vi "Salman's Tip Tester.vi"() -> ()   [LabVIEW 2016]
uses:
  <instrlib>/Stanford Research 830/Public/Data/Read (All Parameters).vi
  <vilib>/Analysis/1siggen.llb/Ramp Pattern by Delta.vi
  <vilib>/express/express shared/transition.llb/Dynamic To Waveform Array.vi
  <vilib>/express/express signal manip/GetorSetDDTAttributes/Set DDT Attributes/SetT0.vi
  <vilib>/express/express shared/transition.llb/Waveform Array To Dynamic.vi
  <vilib>/express/express signal manip/GetorSetDDTAttributes/Set DDT Attributes/Set DDT Properties.xnode
  <vilib>/Analysis/NI_AALBase.lvlib
  <instrlib>/Stanford Research 830/Stanford Research 830.lvlib
  <instrlib>/Agilent 3352X Series/Agilent 3352X Series.lvlib
panel:
  out "Reference Frequency":dbl
  in  "stop":bool
  out "Y-Value":dbl
  out "X-Value":dbl
  in  "?":T1(tab)
  in  "Lock In":refnum<visa-resource-name>
  in  "Frequency Generator":refnum<visa-resource-name>
  in  "Sensitivity":i16(ring)=-1 items=["Auto Gain"=-1, "2 nV/fA"=0, "5 nV/fA"=1, "10 nV/fA"=2, "20 nV/fA"=3, "50 nV/fA"=4, "100 nV/fA"=5, "200 nV/fA"=6, "500 nV/fA"=7, "1 uV/pA"=8, "2 uV/pA"=9, "5 uV/pA"=10, "10 uV/pA"=11, "20 uV/pA"=12, "50 uV/pA"=13, "100 uV/pA"=14, "200 uV/pA"=15, "500 uV/pA"=16, "1 mV/nA"=17, "2 mV/nA"=18, "5 mV/nA"=19, "10 mV/nA"=20, "20 mV/nA"=21, "50 mV/nA"=22, "100 mV/nA"=23, "200 mV/nA"=24, "500 mV/mA"=25, "1 V/uA"=26]
  in  "Auto Phase":bool=TRUE
  in  "Lock In Frequency (Hz)":dbl=1000.0
  in  "Lock In Output (V)":dbl=1.0
  in  "External Reference Trigger":u16(ring) items=["Sine Zero Crossing", "TTL Rising Edge", "TTL Falling Edge"]
  in  "Reference Source":u16(ring)=1 items=["External", "Internal"]
  in  "Amplitude (V)":dbl=0.1
  in  "Waveform Function":i32(ring) items=["Sine"=0, "Square"=1, "Ramp"=2, "Noise"=3, "DC"=4, "Triangle"=5, "Pulse"=6, "Sinc"=11, "D-Lorentz"=12, "Gaussian"=13, "Expo Fall"=14, "Expo Rise"=15, "Haversine"=16]
  in  "Frequency (Hz)":dbl=1000.0
  in  "Save File Name":path=path "G:/UCB/Instruments/tip making/Qplus AFM tip making/qplus test/Caihong/CJ39.xlsx" caption="Filename"
  out "Frequency (Hz) 2":dbl
  out "XY Graph 3":cluster{dbl[], dbl[]}[](graph) caption="XY Graph 2"
  out "XY Graph 2":cluster{dbl[], dbl[]}[](graph)
  in  "Start Sweep":bool
  in  "Wait Time (s)":dbl
  in  "Step Size (Hz)":dbl
  in  "Final Frequency":dbl
  in  "Start Frequency":dbl
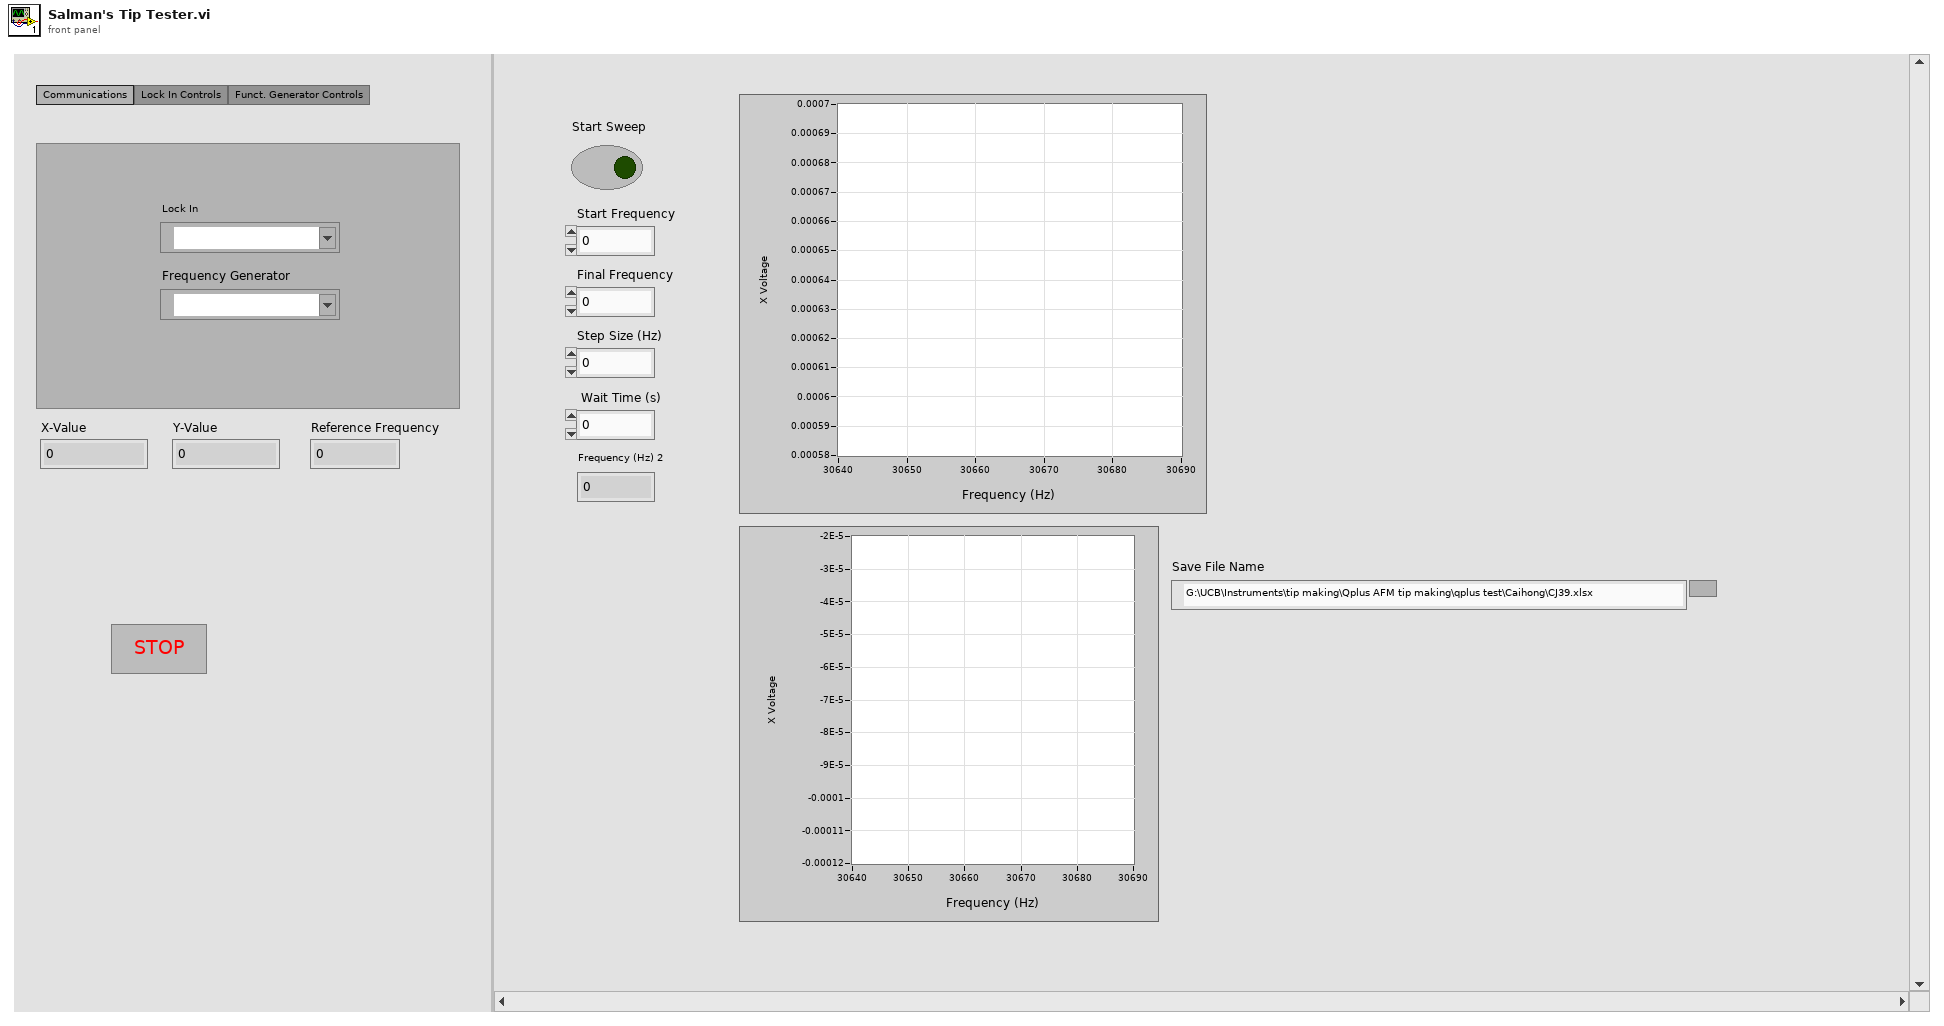
[diagram p1: front panel]
types:
  T1 = enum32{"Communications", "Lock In Controls", "Funct. Generator Controls"}
  T2 = cluster{"X-Value":dbl, "Y-Value":dbl, "R-Value":dbl, "Theta-Value":dbl, "Aux In 1 Value":dbl, "Aux In 2 Value":dbl, "Aux In 3 Value":dbl, "Aux In 4 Value":dbl, "Reference Frequency":dbl, "Channel 1 Display":dbl, "Channel 2 Display":dbl}
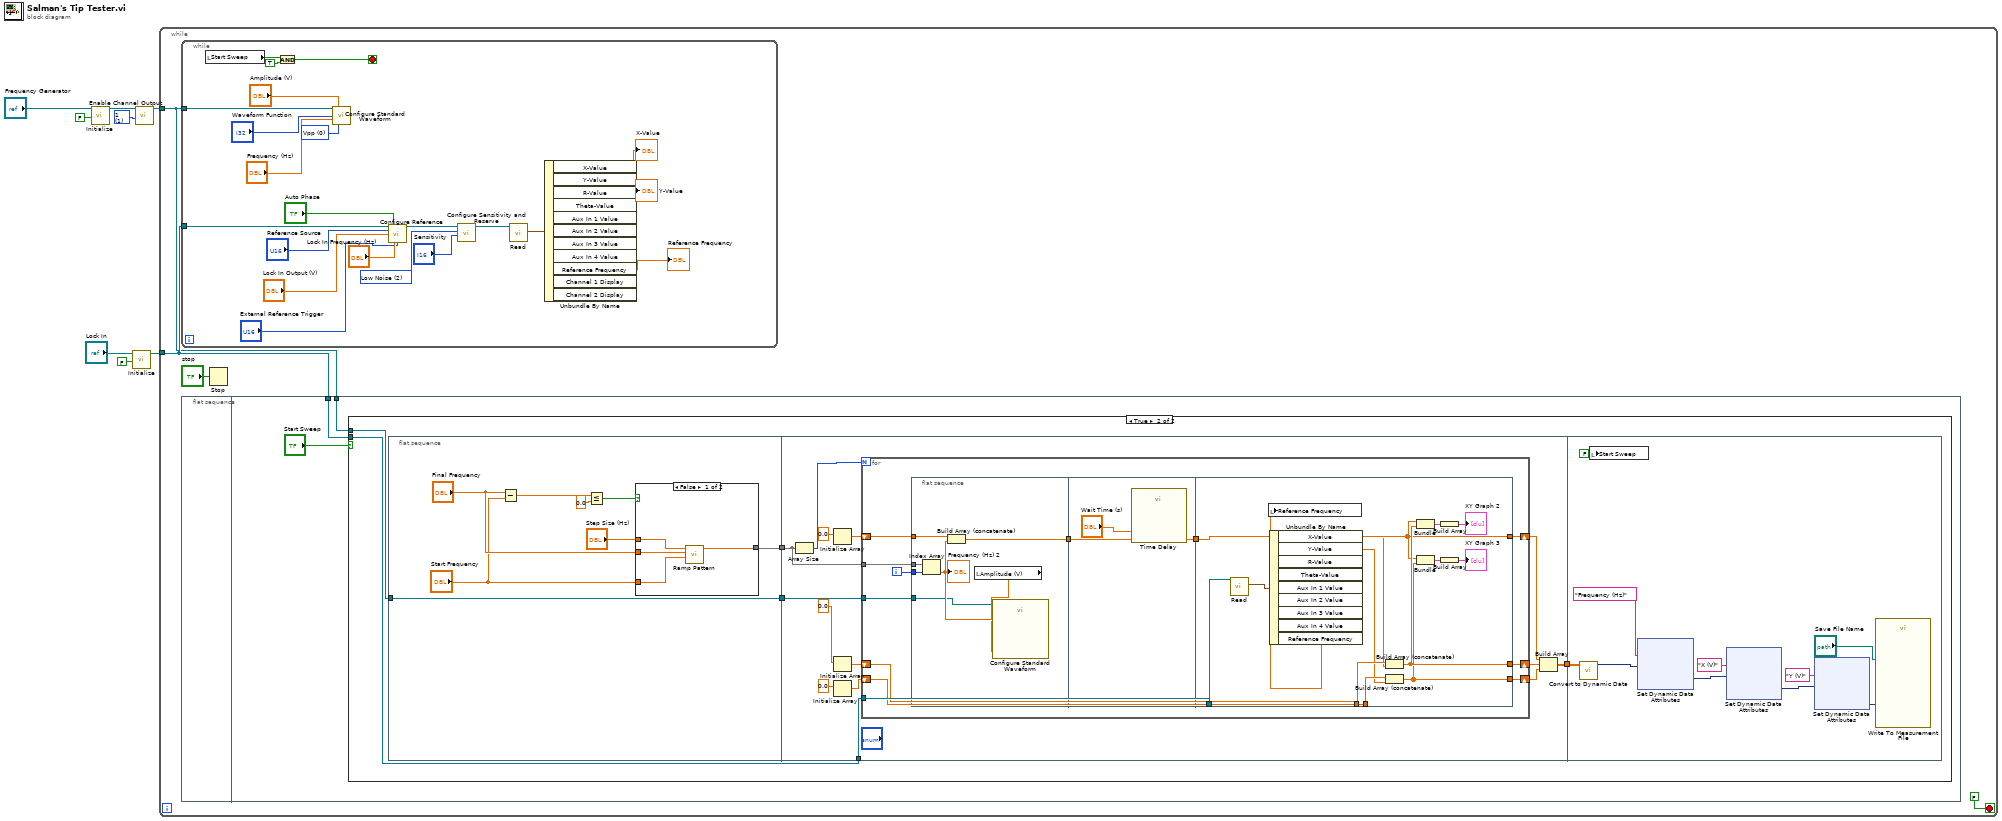
[diagram p0: block diagram]
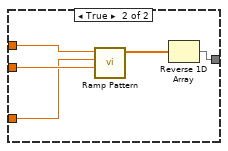
[diagram p3: hidden frame]
diagram:
  w3 = u16 1 items=["1"=1, "2"=2] ("Channel (1: 1)")
  n1 = call <instrlib>:"Initialize.vi"("Reset (Enable)"=FALSE ("Reset (True)"), "VISA resource name"="Frequency Generator") -> ("VISA resource name out"=w2:refnum<visa-resource-name>)  [unwired: 8 in, 1 out]
  n2 = call <instrlib>:"Initialize.vi"("Reset (True)"=FALSE, "VISA resource name"="Lock In") -> ("VISA resource name out"=w7:refnum<visa-resource-name>)  [unwired: 8 in, 1 out]
  n3 = call <instrlib>:"Enable Channel Output.vi"("Channel (1: 1)"=w3, "VISA resource name"=w2) -> ("VISA resource name out"=w1:refnum<visa-resource-name>)  [unwired: 8 in, 1 out]
  n4 = while {
    tunnel: w7 -> [w12]
    tunnel: w1 -> [w9]
    stop <- FALSE stop-if-true
    n5 = while {
      tunnel: w12 -> [w160]
      tunnel: w9 -> [w143]
      stop <- w154 stop-if-true
      w144 = 0 items=["Vpp", "VRMS", "DBM"] ("Amplitude Unit (0: Vpp)")
      w152 = i16 2 items=["Auto Reserve"=-1, "High Reserve"=0, "Normal"=1, "Low Noise"=2] ("Dynamic Reserve (-1: Auto Reserve)")
      n6 = local read "Start Sweep"() -> (w156:bool)
      n7 = And(x=w156, y=TRUE) -> (x .and. y?=w154:bool)
      n8 = call <instrlib>:"Configure Standard Waveform.vi"("VISA resource name"=w143, "Amplitude (0.1 Vpp)"="Amplitude (V)", "Waveform Function (0: Sine)"="Waveform Function", "Frequency/Sample Rate/Bandwidth (1000 Hz)"="Frequency (Hz)", "Amplitude Unit (0: Vpp)"=w144) -> ()  [unwired: 9 in, 2 out]
      n9 = call "Configure Reference.vi"("VISA resource name"=w160, "Auto Phase (T: Enabled)"="Auto Phase", "Reference Source (1: Internal)"="Reference Source", "Sine Output Amplitude (1 V)"="Lock In Output (V)", "Internal Reference Frequency (1000 Hz)"="Lock In Frequency (Hz)", "External Reference Trigger (0: Sine Zero Crossing)"="External Reference Trigger") -> ("VISA resource name out"=w153:refnum<visa-resource-name>)  [unwired: 8 in, 1 out]
      n10 = call <instrlib>:"Configure Sensitivity and Reserve.vi"("Sensitivity (-1: Auto gain)"="Sensitivity", "Dynamic Reserve (-1: Auto Reserve)"=w152, "VISA resource name"=w153) -> ("VISA resource name out"=w150:refnum<visa-resource-name>)  [unwired: 7 in, 1 out]
      n11 = call-poly <instrlib>:"Read.vi"("VISA resource name"=w150) -> ("Parameter Values"=w142:T2)  [unwired: 8 in, 2 out]
      n12 = Unbundle By Name(w142) -> ("X-Value"=→"X-Value":dbl, "Y-Value"=→"Y-Value":dbl, "Reference Frequency"=→"Reference Frequency":dbl)  [unwired: 8 out]
    }
    n13 = flat-sequence {
      tunnel: w12 -> [w14]
      tunnel: w9 -> [w13]
      frame #0 {
      }
      frame #1 {
        n14 = case shown="True" "Start Sweep" {
          tunnel: w14 -> [_ w19]
          tunnel: w13 -> [_ w18]
          frame False {
          }
          frame True {
            n15 = flat-sequence {
              tunnel: [w23] -> w20
              tunnel: w18 -> [w21]
              tunnel: [w21] -> w17
              tunnel: w20 -> [w51]
              tunnel: w19 -> [w47]
              tunnel: w17 -> [w44]
              tunnel: [w38] -> w16
              tunnel: w16 -> [w95]
              frame #0 {
                n16 = Subtract(x="Final Frequency", y="Start Frequency") -> (x-y=w28:dbl)
                n17 = Less Or Equal?(x=w28, y=0.0) -> (x <= y?=w26:bool)
                n18 = case shown="False" w26 {
                  tunnel: "Final Frequency" -> [w32 w34]
                  tunnel: "Start Frequency" -> [w31 w33]
                  tunnel: "Step Size (Hz)" -> [w30 w37]
                  tunnel: [w29 w35] -> w23
                  frame False {
                    n19 = call-poly <vilib>:"Ramp Pattern.vi"("start"=w31, "end"=w32, "delta"=w30) -> ("Ramp Pattern"=w29:dbl[])  [unwired: 6 in, 2 out]
                  }
                  frame True {
                    n20 = call-poly <vilib>:"Ramp Pattern.vi"("start"=w34, "end"=w33, "delta"=w37) -> ("Ramp Pattern"=w36:dbl[])  [unwired: 6 in, 2 out]
                    n21 = Reverse 1D Array(array=w36) -> (reversed array=w35:dbl[])
                  }
                }
              }
              frame #1 {
                n22 = Array Size(array=w51) -> (size(s)=w49:i32)
                n23 = Initialize Array(0.0 ("element")) -> (w48:dbl[])  [unwired: 1 in]
                n24 = Initialize Array(0.0 ("element")) -> (w45:dbl[])  [unwired: 1 in]
                n25 = Initialize Array(0.0 ("element")) -> (w42:dbl[])  [unwired: 1 in]
                n26 = for {
                  N: w49 -> [_]
                  tunnel: w51 -> [w61]
                  shift-right: [w60] -> w39
                  shift-left: w48 -> [w63]
                  tunnel: w47 -> [w57]
                  shift-right: [w56] -> w41
                  shift-left: w45 -> [w55]
                  tunnel: w44 -> [w54]
                  shift-right: [w52] -> w40
                  shift-left: w42 -> [w53]
                  i -> [w62]
                  n27 = flat-sequence {
                    tunnel: w63 -> [w70]
                    tunnel: w62 -> [w69]
                    tunnel: w61 -> [w68]
                    tunnel: [w67] -> w58
                    tunnel: w54 -> [w64]
                    tunnel: [w71] -> w59
                    tunnel: w58 -> [w71]
                    tunnel: [w76] -> w60
                    tunnel: w59 -> [w76]
                    tunnel: w57 -> [w74]
                    tunnel: w55 -> [w85]
                    tunnel: [w84] -> w56
                    tunnel: w53 -> [w81]
                    tunnel: [w77] -> w52
                    frame #0 {
                      n28 = Index Array(array=w68, index=w69) -> (element=w66:dbl)
                      "Frequency (Hz) 2" <- w66
                      n29 = Build Array (concatenate)(w70, w66) -> (w67:dbl[])
                      n30 = local read "Amplitude (V)"() -> (w65:dbl)
                      n31 = call <instrlib>:"Configure Standard Waveform.vi"("VISA resource name"=w64, "Amplitude (0.1 Vpp)"=w65, "Frequency/Sample Rate/Bandwidth (1000 Hz)"=w66) -> ()  [unwired: 11 in, 2 out]
                    }
                    frame #1 {
                      n32 = call "Time Delay"("Delay Time (s)"="Wait Time (s)") -> ()  [unwired: 10 in, 1 out]
                    }
                    frame #2 {
                      n33 = call-poly <instrlib>:"Read.vi"("VISA resource name"=w74) -> ("Parameter Values"=w82:T2)  [unwired: 8 in, 2 out]
                      n34 = Unbundle By Name(w82) -> ("X-Value"=w75:dbl, "Y-Value"=w80:dbl, "Reference Frequency"=w73:dbl)  [unwired: 6 out]
                      n35 = local write "Reference Frequency"(w73) -> ()
                      n36 = Build Array (concatenate)(w85, w75) -> (w84:dbl[])
                      n37 = Build Array (concatenate)(w81, w80) -> (w77:dbl[])
                      n38 = Bundle(w76, w84) -> (w86:cluster{dbl[], dbl[]})  [unwired: 1 in]
                      n39 = Bundle(w76, w77) -> (w79:cluster{dbl[], dbl[]})  [unwired: 1 in]
                      n40 = Build Array(w86) -> (→"XY Graph 2":cluster{dbl[], dbl[]}[])
                      n41 = Build Array(w79) -> (→"XY Graph 3":cluster{dbl[], dbl[]}[])
                    }
                  }
                }
                n42 = Build Array(w39, w41, w40) -> (w38:dbl[][])
              }
              frame #2 {
                n43 = call "Convert to Dynamic Data"("2D Array"=w95) -> ("Dynamic Data Type"=w94:dynamicdata)  [unwired: 3 in]
                n44 = local write "Start Sweep"(FALSE) -> ()
                n45 = xnode ("Set Dynamic Data Attributes")("Signals In"=w94, "Signal Name"="Frequency (Hz)") -> ("Signals Out"=w89:dynamicdata)  [unwired: 2 in, 1 out]
                n46 = xnode ("Set Dynamic Data Attributes")("Signals In"=w89, "Signal Name"="X (V)") -> ("Signals Out"=w88:dynamicdata)  [unwired: 2 in, 1 out]
                n47 = xnode ("Set Dynamic Data Attributes")("Signals In"=w88, "Signal Name"="Y (V)") -> ("Signals Out"=w92:dynamicdata)  [unwired: 2 in, 1 out]
                n48 = call "Write To Measurement File"("Signals"=w92, "Filename"="Save File Name") -> ()  [unwired: 15 in, 3 out]
              }
            }
          }
        }
      }
    }
    n49 = Stop(stop? (T)="stop") -> ()
  }
